vi "XY Go.vi"(8 "error in (no error)":errorcluster, 9 "Speed":dbl, 10 "XY":dbl[](array[numeric]), 11 "Gantry in":refnum<class "A3200.lvclass">) -> (0 "error out":errorcluster, 3 "Gantry out":refnum<class "A3200.lvclass">)   [LabVIEW 2016, in "A3200.lvclass"]
uses:
  A3200.lvclass
  A3200.lvclass/A3200.ctl
  <userlib>/Aerotech A3200.lnk/Aerotech VIs.lvlib
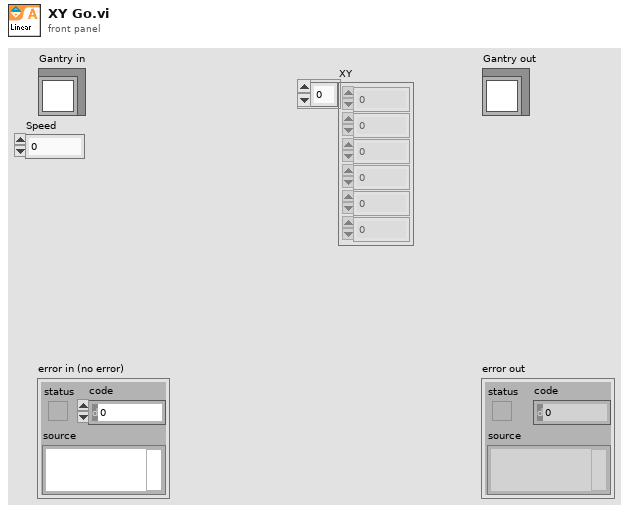
[diagram p1: front panel]
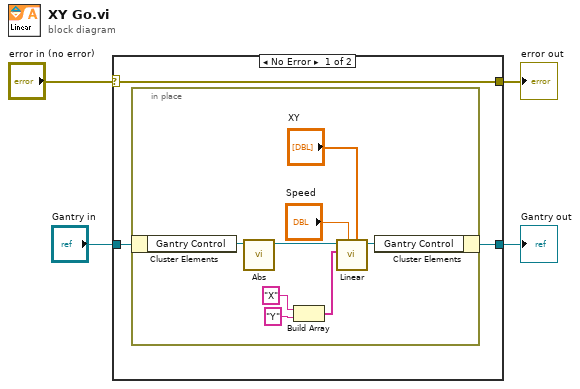
[diagram p0: block diagram]
diagram:
  n1 = case shown="No Error" "error in (no error)" {
    selector: "error in (no error)" -> [w7 w17]
    tunnel: [w7 w17] -> w3
    tunnel: [w6 w16] -> w2
    tunnel: "Gantry in" -> [w5 w16]
    frame No Error {
      n2 = in-place {
        n3 = in-place-cluster #1(w5) -> ("Gantry Control"=w10:refnum<k24>)
        n4 = call <userlib>:"Abs.vi"("controller in"=w10) -> ("controller out"=w9:refnum<k24>)  [unwired: 9 in, 1 out]
        n5 = Build Array("X" ("format string"), "Y" ("format string")) -> (w13:string[])
        n6 = call <userlib>:"Linear.vi"("distances"="XY", "speed"="Speed", "axis names"=w13, "controller in"=w9) -> ("controller out"=w11:refnum<k24>)  [unwired: 6 in, 1 out]
        n7 = in-place-cluster #1("Gantry Control"=w11) -> (w6:refnum<class "A3200.lvclass">)
      }
    }
    frame Error {
    }
  }
  "error out" <- w3
  "Gantry out" <- w2
